vi "vision distance.vi"(11 "Image width":dbl) -> (3 "Distance":dbl)   [LabVIEW 2015]
uses:
  cogs.vi
panel:
  out "alpha":dbl
  in  "right":dbl
  in  "left":dbl
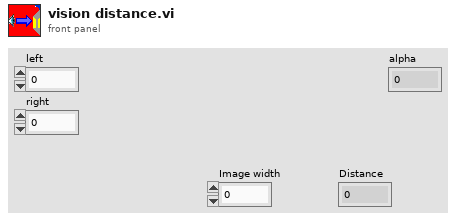
[diagram p1: front panel]
types:
  T1 = cluster{"Global Rectangle":cluster{"x1Left":i32, "y1Top":i32, "x2Right":i32, "y2Bottom":i32}, "Centroid":cluster{"x":sgl, "y":sgl}, "Object Size":u32, "Score":dbl}
  T2 = cluster{"x1Left":i32, "y1Top":i32, "x2Right":i32, "y2Bottom":i32}
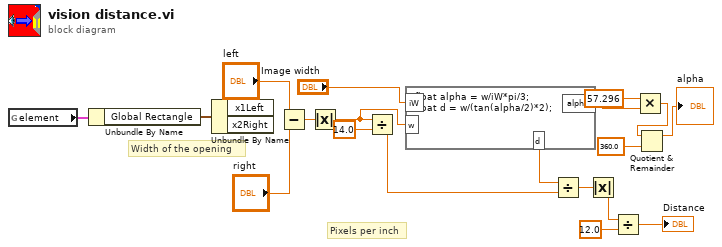
[diagram p0: block diagram]
diagram:
  # "Pixels per inch"
  # "Width of the opening"
  n1 = global read "cogs.vi" "element"() -> (w19:T1)
  n2 = Unbundle By Name(w19) -> ("Global Rectangle"=w18:T2)
  n3 = Unbundle By Name(w18) -> ()  [unwired: 2 out]
  n4 = Subtract(x="left", y="right") -> (x-y=w17:dbl)
  n5 = Absolute Value(x=w17) -> (abs(x)=w10:dbl)
  n6 = Divide(x=w10, y=14.0) -> (x/y=w8:dbl)
  n7 = formula code="float alpha = w/iW*pi/3;\nfloat d = w/(tan(alpha/2)*2);"("w"=w10, "iW"="Image width") -> ("d"=w9:dbl, "alpha"=w13:dbl)
  n8 = Divide(x=w9, y=w8) -> (x/y=w7:dbl)
  n9 = Absolute Value(x=w7) -> (abs(x)=w3:dbl)
  n10 = Divide(x=w3, y=12.0) -> (x/y=→"Distance":dbl)
  n11 = Multiply(x=57.296, y=w13) -> (x*y=w5:dbl)
  n12 = Quotient & Remainder(x=w5, y=360.0) -> (x-y*floor(x/y)=→"alpha":dbl)  [unwired: 1 out]
